vi "Write Data.vi"(8 "error in (no error)":errorcluster, 9 "Value":u8 format="%.0x", 11 "Grove I2C LCD in":refnum<class "Grove I2C LCD.lvclass">) -> (0 "error out":errorcluster, 3 "Grove I2C LCD out":refnum<class "Grove I2C LCD.lvclass">)   [LabVIEW 2020, in "CTI-Peripheral.lvlib" / "Grove I2C LCD.lvclass"]
uses:
  Grove I2C LCD.lvclass
  Grove I2C LCD.lvclass/Grove I2C LCD.ctl
  CTI/I2C Connection/I2C Connection.lvclass/I2C Connection.ctl
  CTI/I2C Connection/I2C Connection.lvclass
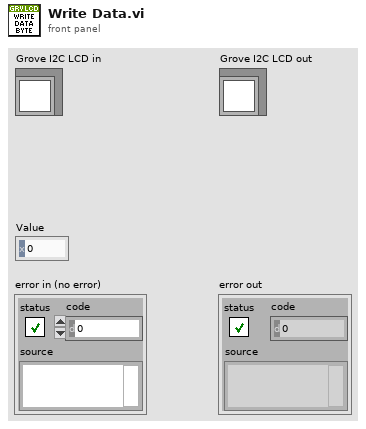
[diagram p1: front panel]
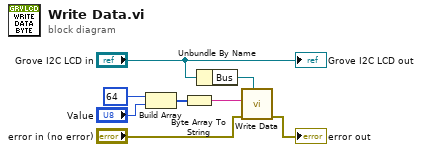
[diagram p0: block diagram]
diagram:
  n1 = Build Array(u8 64 ("Value"), "Value") -> (w6:u8[])
  n2 = Byte Array To String(unsigned byte array=w6) -> (string=w5:string)
  n3 = Unbundle By Name("Grove I2C LCD in") -> ("Bus"=w8:refnum<class "I2C Connection.lvclass">)
  n4 = call "Write Data.vi"("I2C Peripheral"=w8, "error in (no error)"="error in (no error)", "Data"=w5) -> ("error out"=→"error out":errorcluster)  [unwired: 8 in]
  "Grove I2C LCD out" <- "Grove I2C LCD in"
